vi "Delete Device.vi"(8 "error in":errorcluster, 9 "variant":variant) -> (0 "error out":errorcluster)   [LabVIEW 2024, in "Data Base.lvlib"]
uses:
  Data Base.lvlib
  <vilib>/Utility/config.llb/NI_LVConfig.lvlib
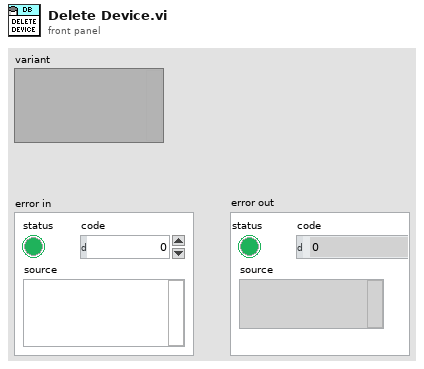
[diagram p1: front panel]
types:
  T1 = typedef "NI_LVConfig.lvlib/Config Data RefNum.ctl" = refnum<k1>
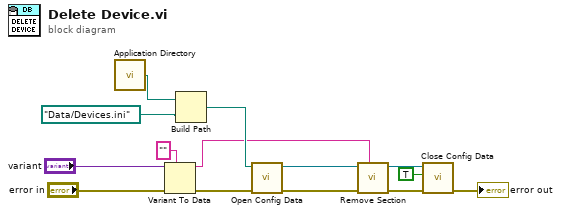
[diagram p0: block diagram]
diagram:
  n1 = call <vilib>:"Application Directory.vi"() -> ("Application Directory"=w12:path)
  n2 = Variant To Data(error in="error in", type="", Variant="variant") -> (data=w3:string, error out=w9:errorcluster)
  n3 = Build Path(base path=w12, name or relative path=path "Data/Devices.ini") -> (appended path=w14:path)
  n4 = call <vilib>:"Open Config Data.vi"("error in (no error)"=w9, "configuration file path"=w14) -> ("error out"=w6:errorcluster, "refnum"=w7:T1)  [unwired: 7 in, 1 out]
  n5 = call <vilib>:"Remove Section.vi"("section"=w3, "error in (no error)"=w6, "refnum"=w7) -> ("error out"=w4:errorcluster, "refnum out"=w5:T1)  [unwired: 6 in, 1 out]
  n6 = call <vilib>:"Close Config Data.vi"("error in (no error)"=w4, "write file if changed (T)"=TRUE, "refnum"=w5) -> ("error out"=→"error out":errorcluster)  [unwired: 7 in, 1 out]
